vi "Setup AWG and Measure Capacitance Only.vi"(4 "cleanup script":string="BeamsOff", 5 "setup script":string="PullDown41v", 6 "error in (no error)":errorcluster, 7 "VNAs Measurement Parameters":T1, 8 "Measurement Id":string="CMax", 9 "Semiconductor Module Context":T2) -> (0 "error out":errorcluster, 3 "Semiconductor Module Context Out":T2)   [LabVIEW 2013]
uses:
  <vilib>/NI_TestStand_SemiconductorModule/NI_TestStand_Semiconductor_Module.lvlibp/PinMap/General/SemiconductorModuleContext.ctl
  VNA/VNAs Measurement Parameters.ctl
  <instrlib>/niHSDIO/niHSDIO.llb/niHSDIO_ctl Trigger Script - trigID Values (Ring).ctl
  <vilib>/NI_TestStand_SemiconductorModule/NI_TestStand_Semiconductor_Module.lvlibp
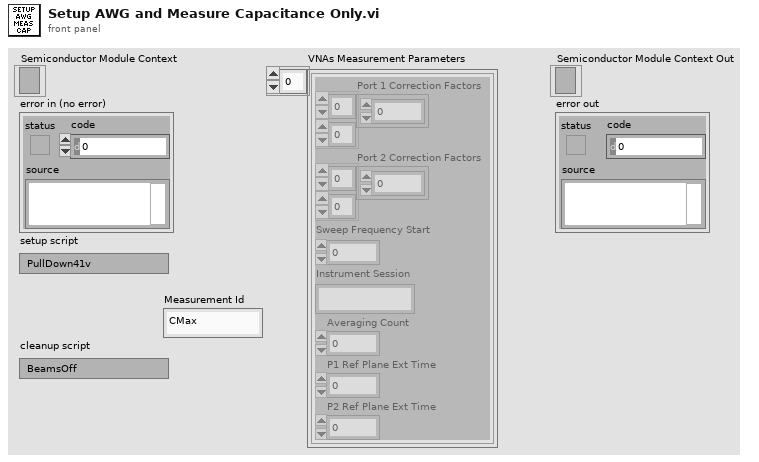
[diagram p1: front panel]
types:
  T1 = typedef "VNAs Measurement Parameters.ctl" = cluster{"Port 1 Correction Factors":cdb[][], "Port 2 Correction Factors":cdb[][], "Sweep Frequency Start":dbl, "Instrument Session":string, "Averaging Count":i32, "P1 Ref Plane Ext Time":dbl, "P2 Ref Plane Ext Time":dbl}[]
  T2 = typedef "NI_TestStand_Semiconductor_Module.lvlibp/SemiconductorModuleContext.ctl" = refnum<k7>
  T3 = typedef "niHSDIO_ctl Trigger Script - trigID Values (Ring).ctl" = string
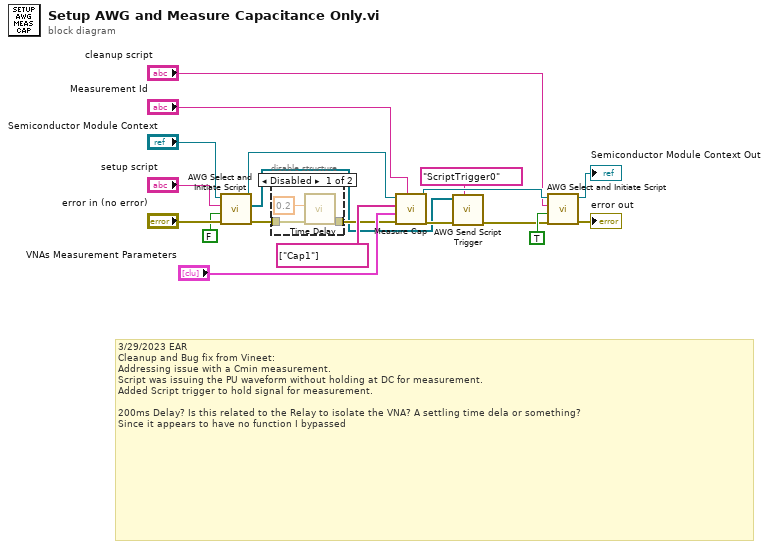
[diagram p0: block diagram]
diagram:
  # "3/29/2023 EAR\nCleanup and Bug fix from Vineet:\nAddressing issue with a Cmin measurement.\nScript was issuing the PU waveform without holding at DC for measurement.\nAdded Script trigger to hold signal for measurement.\n\n200ms Delay? Is this related to the Relay to isolate the VNA? A settling time dela or something?\nSince it appears to have no function I bypassed"
  n1 = call "AWG Select and Initiate Script.vi"("error in (no error)"="error in (no error)", "Wait for Completion"=FALSE, "script name"="setup script", "Semiconductor Module Context"="Semiconductor Module Context") -> ("error out"=w15:errorcluster, "Sessions Out"=w1:refnum<k15>[], "Semiconductor Module Context Out"=w11:T2)  [unwired: 5 in]
  n2 = disable-structure shown="Disabled" {
    disable-tunnel: w15 -> [w21 w23]
    disable-tunnel: [w20 w23] -> w4
    frame Disabled {
      n3 = call "Time Delay"("error in (no error)"=w21, "Delay Time (s)"=0.2) -> ("error out"=w20:errorcluster)  [unwired: 9 in]
    }
    frame Enabled {
    }
  }
  n4 = call "Measure Cap.vi"("Measurement Id"="Measurement Id", "error in (no error)"=w4, "VNAs Measurement Parameters"="VNAs Measurement Parameters", "Pins"=string[] ["Cap1"] ("Capacitance Pins"), "Semiconductor Module Context"=w11) -> ("error out"=w3:errorcluster, "Semiconductor Module Context Out"=w12:T2)  [unwired: 4 in, 1 out]
  n5 = call "AWG Send Script Trigger.vi"("trigger id (script trigger 0)"=T3 "ScriptTrigger0", "error in (no error)"=w3, "AWG Sessions In"=w1) -> ("error out"=w2:errorcluster)  [unwired: 7 in, 1 out]
  n6 = call "AWG Select and Initiate Script.vi"("error in (no error)"=w2, "Wait for Completion"=TRUE, "script name"="cleanup script", "Semiconductor Module Context"=w12) -> ("error out"=→"error out":errorcluster, "Semiconductor Module Context Out"=→"Semiconductor Module Context Out":T2)  [unwired: 5 in, 1 out]
